vi "Power monitor main.vi"(8 "Mailbox to TOP":T2, 11 "Module mailbox":T2) -> (0 "stop":bool)   [LabVIEW 2024, in "Power monitor.lvlib"]
doc: "This example demonstrates how to get the power source status of your computer. This VI constantly polls the operating system for the power source information. The power source values are an estimate provided by the battery driver. This VI was developed for use in laptop computers, however it also operates correctly in UPS units with a Windows battery driver. The return values of the call to the Windows DLL are formatted and presented in the front panel. \n\nThis example requires Windows 98/2000/NT/XP.\n\nModified by PBrooks, 21 Sept 2006; original from \nhttp://sine.ni.com/apps/utf8/niepd_web_display.display_epd4?p_guid=DA42328FD16D1FDCE034080020E74861"
uses:
  Power monitor.lvlib
  Messenger service/Data types/Module name.ctl
  Messenger service/MessengerLib.lvlib
  PwrM commands.ctl
  PwrM status.ctl
  Messenger service/Data types/Mailbox address.ctl
panel:
  out "UPS status":T1 {"Last update" format="%<%H:%M:%S>T"}
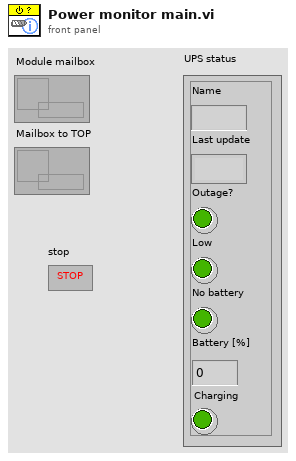
[diagram p1: front panel]
types:
  T1 = typedef "Power monitor.lvlib/PwrM status.ctl" = cluster{"Name":string, "Last update":timestamp, "Outage?":bool, "Low":bool, "No battery":bool, "Battery [%]":u8, "Charging":bool}
  T2 = typedef "MessengerLib.lvlib/Mailbox address.ctl" = refnum<queue>
  T3 = typedef "SystemPowerStatus.ctl" = cluster{"ACLineStatus":u8, "BatteryFlag":u8, "BatteryLifePercent":u8, "Reserved":u8, "BatteryLifeTime":i32, "BatteryFullLifeTime":i32}
  T4 = typedef "Module name.ctl" = enum16{"Emty", "Magnet", "VTI", "Excitation", "Servo", "Acquisition", "Rotator", "Digitizer", "SMU2450", "Carousel", "Multimeter", "Tmp monitor", "Power monitor"}
  T5 = typedef "Power monitor.lvlib/PwrM commands.ctl" = enum16{"Ignore", "Update", "End"}
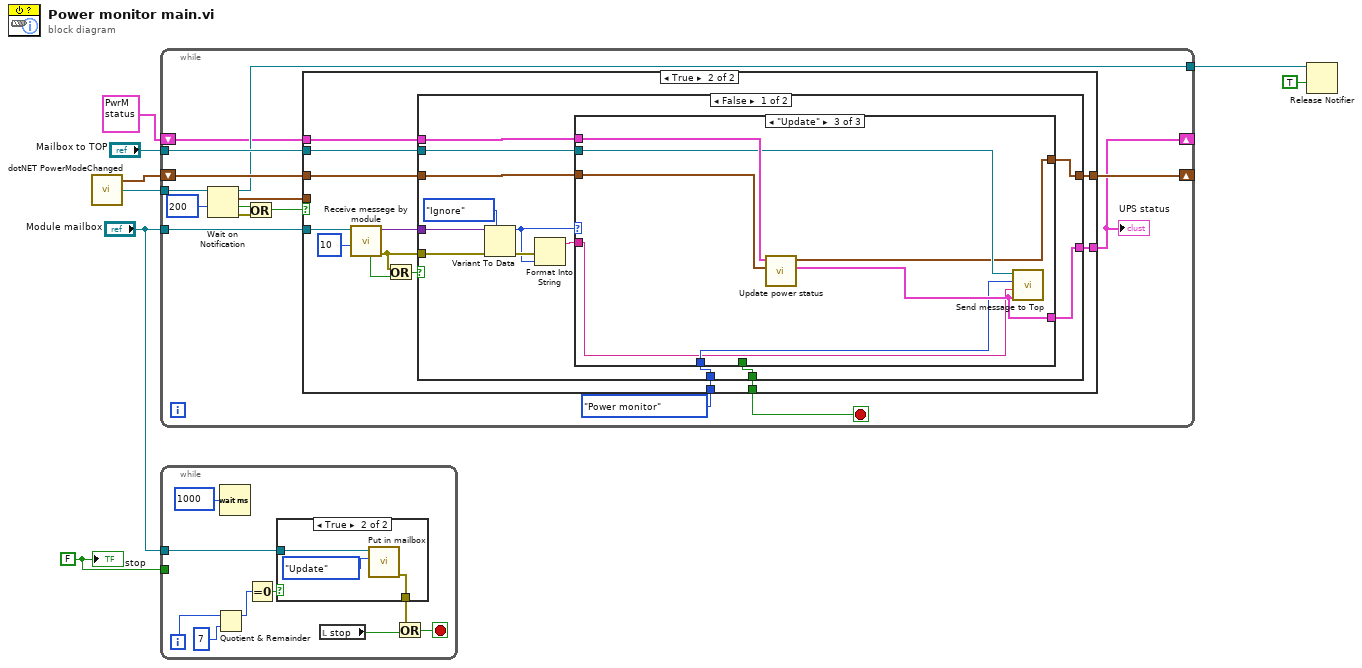
[diagram p0: block diagram]
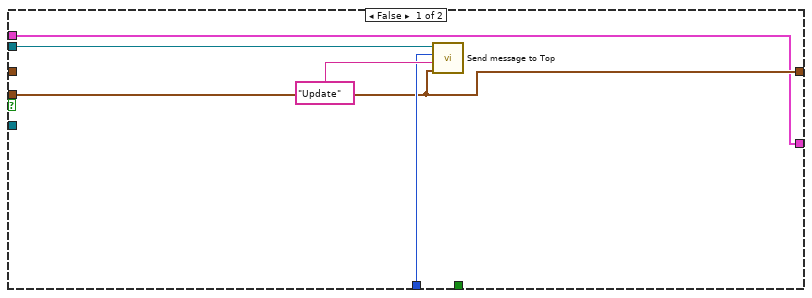
[diagram p3: hidden frame]
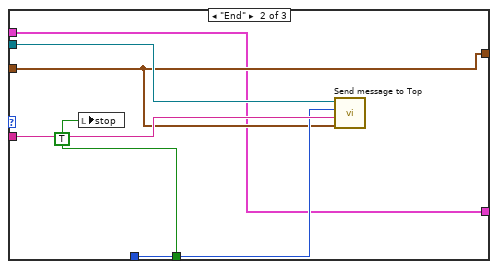
[diagram p5: hidden frame]
diagram:
  w5 = FALSE ("stop")
  n1 = call "dotNET PowerModeChanged.vi"() -> ("PowerModeChanged Notifier"=w7:refnum<notifier>, "SystemPowerStatus"=w4:T3)  [unwired: 4 in]
  n2 = while {
    tunnel: "Mailbox to TOP" -> [w14]
    tunnel: "Module mailbox" -> [w18]
    tunnel: w7 -> [w20]
    shift-right: [w16] -> _
    shift-left: w4 -> [w15]
    tunnel: [w11] -> w3
    shift-right: [w10] -> _
    shift-left: T1 {"Name"="", "Last update"=timestamp(0 s since 1904-01-01), "Outage?"=FALSE, "Low"=FALSE, "No battery"=FALSE, "Battery [%]"=0, "Charging"=FALSE} ("UPS status") -> [w9]
    stop <- w12 stop-if-true
    n3 = Wait on Notification(notifier=w20, timeout in ms (-1)=200) -> (notifier out=w11:refnum<notifier>, notification=w17:T3, timed out?=w22:bool, error out=w23:errorcluster)  [unwired: 2 in]
    n4 = Or(x=w22, y=w23) -> (x .or. y?=w19:bool)
    n5 = case shown="True" w19 {
      tunnel: w18 -> [_ w40]
      tunnel: w17 -> [w26 _]
      tunnel: [w26 w39] -> w16
      tunnel: w15 -> [_ w38]
      tunnel: w14 -> [w25 w34]
      tunnel: Module_name."Power monitor" ("Module") -> [w27 w33]
      tunnel: [_ w32] -> w12
      tunnel: [w24 w30] -> w10
      tunnel: w9 -> [w24 w29]
      frame False {
        n6 = call "Send message to Top.vi"("Data"=w26, "Response"="Update", "Module"=w27, "Mailbox address in"=w25) -> ()  [unwired: 6 in, 2 out]
      }
      frame True {
        n7 = call "Receive messege by module.vi"("timeout in ms (-1)"=10, "Module mailbox"=w40) -> ("error out"=w36:errorcluster, "Data"=w31:variant, "timed out?"=w35:bool)  [unwired: 5 in, 2 out]
        n8 = Or(x=w36, y=w35) -> (x .or. y?=w37:bool)
        n9 = case shown="False" w37 {
          tunnel: w36 -> [w54 _]
          tunnel: [w42 w71] -> w39
          tunnel: w38 -> [w52 w71]
          tunnel: w34 -> [w50 _]
          tunnel: w33 -> [w51 _]
          tunnel: [w46 _] -> w32
          tunnel: w31 -> [w45 _]
          tunnel: [w43 w70] -> w30
          tunnel: w29 -> [w44 w70]
          frame False {
            n10 = Variant To Data(error in=w54, type=PwrM_commands."Ignore", Variant=w45) -> (data=w48:T5, error out=w49:errorcluster)
            n11 = Format Into String(error in=w49, w48) -> (resulting string=w47:string)  [unwired: 2 in, 1 out]
            n12 = case shown="\"Update\"" w48 {
              tunnel: w52 -> [w55 w58 w66]
              tunnel: w51 -> [_ w60 w64]
              tunnel: w50 -> [_ w61 w68]
              tunnel: w47 -> [_ w62 w63]
              tunnel: [_ w59 _] -> w46
              tunnel: w44 -> [w56 w57 w69]
              tunnel: [w56 w57 w67] -> w43
              tunnel: [w55 w58 w65] -> w42
              frame "Ignore", Default {
              }
              frame "End" {
                w59 = TRUE
                n13 = local write "stop"(w59) -> ()
                n14 = call "Send message to Top.vi"("Data"=w58, "Response"=w62, "Module"=w60, "Mailbox address in"=w61) -> ()  [unwired: 6 in, 2 out]
              }
              frame "Update" {
                n15 = call "Update power status.vi"("SystemPowerStatus in"=w66, "UPS status in"=w69) -> ("UPS status out"=w67:T1, "SystemPowerStatus out"=w65:T3)  [unwired: 7 in, 1 out]
                n16 = call "Send message to Top.vi"("Data"=w67, "Response"=w63, "Module"=w64, "Mailbox address in"=w68) -> ()  [unwired: 6 in, 2 out]
              }
            }
          }
          frame True {
          }
        }
      }
    }
    "UPS status" <- w10
  }
  n17 = while {
    tunnel: w5 -> [_]
    tunnel: "Module mailbox" -> [w80]
    i -> [w75]
    stop <- w79 stop-if-true
    n18 = Quotient & Remainder(x=w75, y=7) -> (x-y*floor(x/y)=w72:i32)  [unwired: 1 out]
    n19 = Wait (ms)(milliseconds to wait=u32 1000) -> ()  [unwired: 1 out]
    n20 = Equal To 0?(x=w72) -> (x = 0?=w73:bool)
    n21 = case shown="True" w73 {
      tunnel: w80 -> [_ w82]
      tunnel: [_ w81] -> w78
      frame False {
      }
      frame True {
        n22 = call "Put in mailbox.vi"("Message"=PwrM_commands."Update", "Queue in"=w82) -> ("error out"=w81:errorcluster)  [unwired: 7 in, 2 out]
      }
    }
    n23 = local read "stop"() -> (w77:bool)
    n24 = Or(x=w78, y=w77) -> (x .or. y?=w79:bool)
  }
  n25 = Release Notifier(notifier=w3, force destroy? (F)=TRUE) -> ()  [unwired: 1 in, 3 out]
  "stop" <- w5
